vi "Do Request.vi"(7 "Processing In":refnum<class "Processing.lvclass">, 11 "Approval in":refnum<class "Approval.lvclass">) -> (0 "error out":errorcluster, 5 "Processing":refnum<class "Processing.lvclass">)   [LabVIEW 2020, in "Summer of LabVIEW.lvlib" / "Approval.lvclass"]
uses:
  Approval.lvclass
  <vilib>/IlluminatedG/IG HTTP Server/HTTP Server/Processing/Processing.lvclass
  <vilib>/IlluminatedG/IG HTTP Server/HTTP Server/Security/Security.lvclass
  Submission DB/Submission DB.lvclass
  <vilib>/IlluminatedG/IG HTTP Server/HTTP Server/Processing/Processing.lvclass/Processing.ctl
  SOL User/SOL User.lvclass
  Approval.lvclass/Approval.ctl
  27921333-a6d9-4ef7-a1e8-564b3ac469df.vi
  88be5f75-02fd-4a44-8f6e-b1c4bebe550e.vi
  829331ca-681c-412f-b695-32c1b29cf155.vi
  1527bb29-3afa-4abb-836d-3fd3d95c894d.vi
  27921333-a6d9-4ef7-a1e8-564b3ac469df.vi/36b1f833-cfc6-44a5-864d-b53e3b32e5c8.vi
  88be5f75-02fd-4a44-8f6e-b1c4bebe550e.vi/9528e9df-aefc-4ce0-9221-106a337fd3b6.vi
  829331ca-681c-412f-b695-32c1b29cf155.vi/9528e9df-aefc-4ce0-9221-106a337fd3b6.vi
  1527bb29-3afa-4abb-836d-3fd3d95c894d.vi/9528e9df-aefc-4ce0-9221-106a337fd3b6.vi
  <vilib>/IlluminatedG/IG HTTP Server/HTTP Server/Values/Get Arg Map.vi
  <vilib>/Utility/error.llb/Error Cluster From Error Code.vi
  <vilib>/IlluminatedG/IG HTTP Utils/HTTP Utils/Response/Response.lvclass
  Submission/Submission.lvclass
  SOL-Server/SOL-Server.lvclass
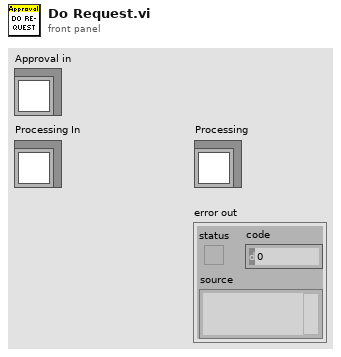
[diagram p1: front panel]
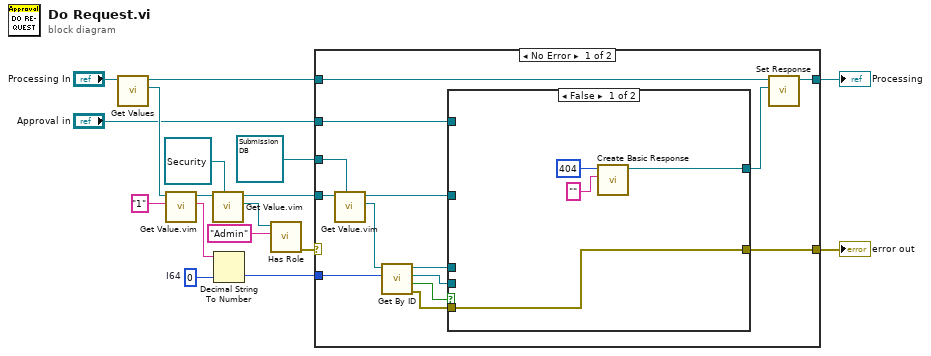
[diagram p0: block diagram]
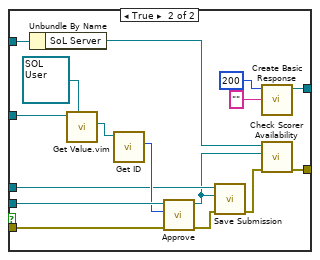
[diagram p2: hidden frame]
diagram:
  w15 = i64 0  # I64
  n1 = call <vilib>:"Get Values.vi"("Processing in"="Processing In") -> ("Values"=w13:refnum<class "Values.lvclass">, "Processing out"=w3:refnum<class "Processing.lvclass">)  [unwired: 9 in]
  n2 = call "Get Value.vim"("Name for Type"="1", "Arguments in"=w13) -> ("Value"=w16:string, "Arguments out"=w12:refnum<class "Values.lvclass">)  [unwired: 7 in, 1 out]
  n3 = call "Get Value.vim"("Type / Server / Service (String)"=refnum<class "Security.lvclass"> refnum ("HTTP Server.lvlib:Security.lvclass"), "Arguments in"=w12) -> ("Value"=w10:refnum<class "Security.lvclass">, "Arguments out"=w8:refnum<class "Values.lvclass">)  [unwired: 7 in, 1 out]
  n4 = Decimal String To Number(string=w16, default (0L)=w15) -> (number=w6:i64)  [unwired: 1 in, 1 out]
  n5 = call <vilib>:"Has Role.vi"("Role"="Admin", "Security in"=w10) -> ("error out"=w7:errorcluster)  [unwired: 7 in, 2 out]
  n6 = case shown="No Error" w7 {
    selector: w7 -> [_ w53]
    tunnel: w8 -> [w31 _]
    tunnel: w6 -> [w30 _]
    tunnel: refnum<class "Submission DB.lvclass"> refnum ("SOL:Submission DB.lvclass") -> [w28 _]
    tunnel: [w20 w53] -> w4
    tunnel: w3 -> [w24 w52]
    tunnel: [w23 w52] -> w2
    tunnel: "Approval in" -> [w19 _]
    frame No Error {
      n7 = call "Get Value.vim"("Type / Server / Service (String)"=w28, "Arguments in"=w31) -> ("Value"=w29:refnum<class "Submission DB.lvclass">, "Arguments out"=w22:refnum<class "Values.lvclass">)  [unwired: 7 in, 1 out]
      n8 = call "Get By ID.vi"("ID"=w30, "Submission DB in"=w29) -> ("error out"=w18:errorcluster, "Found?"=w27:bool, "Submission"=w26:refnum<class "Submission.lvclass">, "Submission DB out"=w21:refnum<class "Submission DB.lvclass">)  [unwired: 6 in]
      n9 = case shown="False" w27 {
        tunnel: w26 -> [_ w51]
        tunnel: [w33 w44] -> w25
        tunnel: w22 -> [_ w50]
        tunnel: w21 -> [_ w46]
        tunnel: [w32 w37] -> w20
        tunnel: w19 -> [_ w41]
        tunnel: w18 -> [w32 w36]
        frame False {
          n10 = call <vilib>:"Create Basic Response.vi"("Payload"="", "Status Code"=u16 404) -> ("Response out"=w33:refnum<class "Response.lvclass">)  [unwired: 8 in, 1 out]
        }
        frame True {
          n11 = Unbundle By Name(w41) -> ("SoL Server"=w40:refnum<class "SOL-Server.lvclass">)
          n12 = call "Get Value.vim"("Type / Server / Service (String)"=refnum<class "SOL User.lvclass"> refnum ("SOL:SOL User.lvclass"), "Arguments in"=w50) -> ("Value"=w48:refnum<class "SOL User.lvclass">)  [unwired: 7 in, 2 out]
          n13 = call "Get ID.vi"("SOL User in"=w48) -> ("ID"=w47:i64)  [unwired: 8 in, 2 out]
          n14 = call "Approve.vi"("error in (no error)"=w36, "Approver ID"=w47, "Submission in"=w51) -> ("error out"=w45:errorcluster, "Submission out"=w39:refnum<class "Submission.lvclass">)  [unwired: 7 in]
          n15 = call "Save Submission.vi"("error in (no error)"=w45, "Submission"=w39, "Submission DB in"=w46) -> ("error out"=w38:errorcluster)  [unwired: 7 in, 1 out]
          n16 = call <vilib>:"Create Basic Response.vi"("Payload"="", "Status Code"=u16 200) -> ("Response out"=w44:refnum<class "Response.lvclass">)  [unwired: 8 in, 1 out]
          n17 = call "Check Scorer Availability.vi"("error in (no error)"=w38, "Submission"=w39, "SOL-Server in"=w40) -> ("error out"=w37:errorcluster)  [unwired: 7 in, 1 out]
        }
      }
      n18 = call <vilib>:"Set Response.vi"("Response"=w25, "Processing in"=w24) -> ("Processing out"=w23:refnum<class "Processing.lvclass">)  [unwired: 9 in]
    }
    frame Error {
      # "No need to do more here, the error returned will trigger the user to login if they aren't (maybe using history or back button after logging out), or if they are logged in but aren't admin, they'll get an error response."
    }
  }
  "error out" <- w4
  "Processing" <- w2
